vi "Find Tests - Error Input - Returns Same Error.vi"() -> ()   [LabVIEW 2017, in "LVUnit Test Discoverer.Tests.lvlib"]
uses:
  LVUnit Test Discoverer.Tests.lvlib
  LVUnit Test Discoverer/LVUnit Test Discoverer.lvclass
  <vilib>/PNR/Transparent Assertions/Transparent Assertions/Transparent Assertions.lvlib
panel:
  out "error out":errorcluster
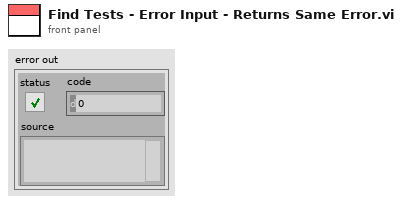
[diagram p1: front panel]
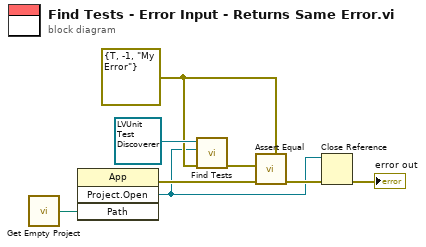
[diagram p0: block diagram]
diagram:
  w3 = errorcluster {"status"=TRUE, "code"=-1, "source"="My Error"} ("error constant")
  n1 = call "Get Empty Project.vi"() -> ("Project File"=w7:path)  [unwired: 2 in]
  n2 = invoke class="App" method="Project.Open"("Path"=w7) -> (error out=w4:errorcluster, "Project:Open"=w1:refnum<vi>)  [unwired: 3 in, 2 out]
  n3 = call-dynamic "Find Tests.vi"("error in (no error)"=w3, "Project Refnum"=w1, "LVUnit Test Discoverer in"=refnum<class "LVUnit Test Discoverer.lvclass"> refnum ("LVUnit Test Discoverer")) -> ("error out"=w5:errorcluster)  [unwired: 6 in, 2 out]
  n4 = call <vilib>:"Assert Equal.vi"("Expected"=w3, "error in (no error)"=w4, "Actual"=w5) -> ("error out"=w6:errorcluster)  [unwired: 8 in]
  n5 = Close Reference(reference=w1, error in (no error)=w6) -> (error out=→"error out":errorcluster)
